vi "Read RX Port.vi"(0 "Refnum in":refnum<k20>, 2 "Timeout (ms)":i32=5000, 5 "Ethernet port":i32, 7 "Elements to Read":u32, 11 "error in (no error)":errorcluster) -> (4 "Refnum out":refnum<k20>, 6 "Data":u8[](array[numeric]), 8 "Elements Remaining out":u32, 15 "error out":errorcluster)   [LabVIEW 2017, in "My Network Host v1.lvlib"]
uses:
  My Network Host v1.lvlib
  <vilib>/Utility/error.llb/Error Cluster From Error Code.vi
  <vilib>/rvi/errors/niLvFpgaAdjustHostInterfaceError.vi
  <vilib>/rvi/interface/nirviMethod/nirviMethod.xnode
  <vilib>/FPGAPlugInAG/Dynamic/niLvFpga_ReadFifo_Dynamic.vi
  <vilib>/rvi/errors/niLvFpgaMergeErrorWithErrorCode.vi
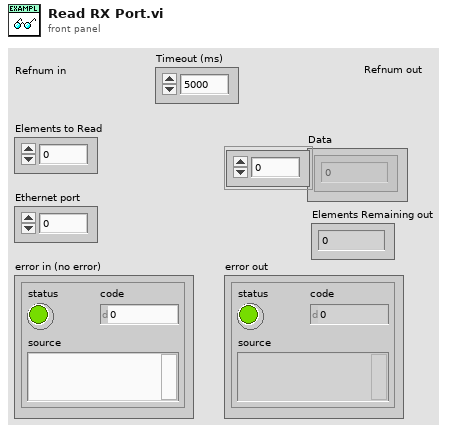
[diagram p1: front panel]
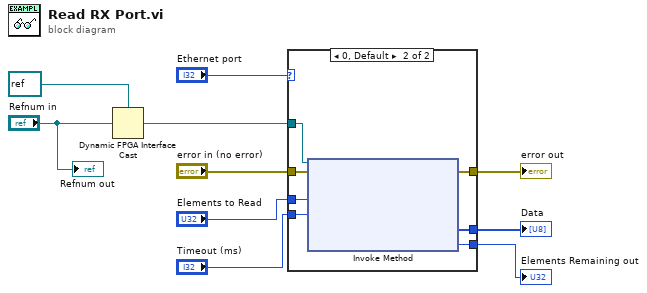
[diagram p0: block diagram]
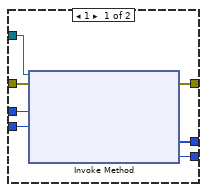
[diagram p2: hidden frame]
diagram:
  n1 = Dynamic FPGA Interface Cast(Session In=refnum<k20> refnum ("Refnum in"), Type="Refnum in") -> (Session Out=w2:refnum<k20>)
  n2 = case shown="0, Default" "Ethernet port" {
    tunnel: w2 -> [w17 w24]
    tunnel: "error in (no error)" -> [w16 w23]
    tunnel: "Elements to Read" -> [w15 w22]
    tunnel: [w14 w21] -> w9
    tunnel: [w13 w20] -> w7
    tunnel: [w12 w19] -> w10
    tunnel: "Timeout (ms)" -> [w11 w18]
    frame 1 {
      n3 = xnode "Invoke Method"("FPGA VI Reference In"=w17, "error in"=w16, "Number of Elements"=w15, "Timeout (ms)"=w11) -> ("error out"=w13:errorcluster, "Data"=w14:u8[], "Elements Remaining"=w12:u32)  [unwired: 1 out]
    }
    frame 0, Default {
      n4 = xnode "Invoke Method"("FPGA VI Reference In"=w24, "error in"=w23, "Number of Elements"=w22, "Timeout (ms)"=w18) -> ("error out"=w20:errorcluster, "Data"=w21:u8[], "Elements Remaining"=w19:u32)  [unwired: 1 out]
    }
  }
  "Elements Remaining out" <- w10
  "Data" <- w9
  "error out" <- w7
  "Refnum out" <- "Refnum in"
